vi "Change FPGA Sample Time.vi"(8 "error in":errorcluster, 11 "tCRD in":refnum<class "Aircraft OPCCRD.lvclass">) -> (0 "error out":errorcluster, 3 "tCRD out":refnum<class "Aircraft OPCCRD.lvclass">)   [LabVIEW 2015, in "Aircraft OPCCRD.lvclass"]
uses:
  Aircraft OPCCRD.lvclass
  Reusable/Instrument/Instrument.lvclass/Instrument.ctl
  Aircraft OPCCRD.lvclass/Aircraft OPCCRD.ctl
  Reusable/Instrument/Read Log Session.vi
  Accessors/Read FPGA Ref.vi
  Reusable/Instrument/Write Restart Requested_.vi
  <vilib>/Utility/error.llb/Error Cluster From Error Code.vi
  <vilib>/rvi/errors/niLvFpgaAdjustHostInterfaceError.vi
  <userlib>/_Session Fwk/Session - Root.lvclass
  tFPGA Ref.ctl
  <vilib>/rvi/interface/nirviReadWriteControl/nirviReadWriteControl.xnode
  FPGA Bitfiles/Aircraft OPCRD Server.lvbitx
  Reusable/Instrument/Instrument.lvclass
  Reusable/Session Log/System Log.lvclass
  NiFpgaLv.dll
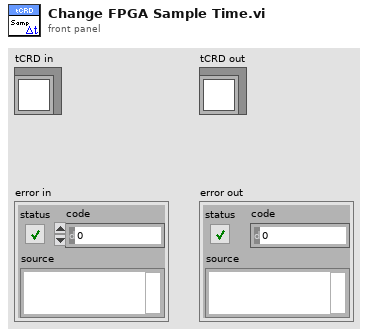
[diagram p1: front panel]
types:
  T1 = typedef "Session - Root.lvclass/Session Handle.ctl" = refnum<data-value>
  T2 = typedef "Aircraft OPCCRD.lvclass/tFPGA Ref.ctl" = refnum<k20>
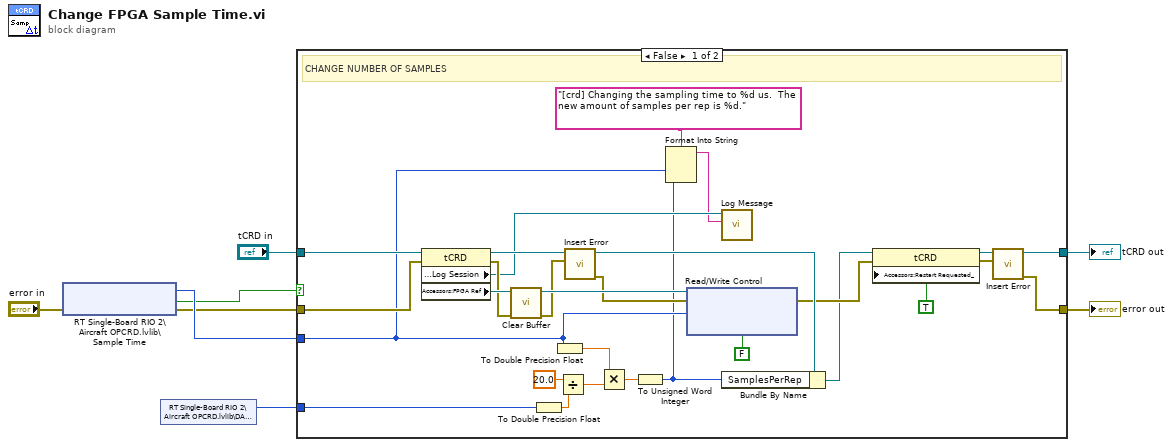
[diagram p0: block diagram]
diagram:
  n1 = shared-variable "RT Single-Board RIO 2\\Aircraft OPCRD.lvlib\\Sample Time"(error in="error in") -> (w8:u16, error out=w5:errorcluster, w2:bool)  [unwired: 1 in]
  n2 = shared-variable "RT Single-Board RIO 2\\Aircraft OPCRD.lvlib\\DAQ Rate"() -> (w1:u8)  [unwired: 1 in, 1 out]
  n3 = case shown="False" w2 {
    tunnel: w5 -> [w15 w38]
    tunnel: "tCRD in" -> [w18 w37]
    tunnel: w8 -> [w12 _]
    tunnel: [w24 w38] -> w6
    tunnel: [w25 w37] -> w3
    tunnel: w1 -> [w33 _]
    frame False {
      # "CHANGE NUMBER OF SAMPLES"
      n4 = property class="tCRD"(reference=w18, error in=w15) -> (reference out=w17:refnum<class "Aircraft OPCCRD.lvclass">, error out=w14:errorcluster, "Accessors:Log Session"=w13:T1, "Accessors:FPGA Ref"=w16:T2)
      n5 = call "Clear Buffer.vi"("error in"=w14, "Refnum in"=w16) -> ("error out"=w28:errorcluster, "FPGA VI Reference Out"=w29:T2)  [unwired: 8 in]
      n6 = To Double Precision Float(number=w33) -> (double precision float=w32:dbl)
      n7 = To Double Precision Float(number=w12) -> (double precision float=w31:dbl)
      n8 = Divide(x=20.0, y=w32) -> (x/y=w35:dbl)
      n9 = call "Insert Error.vi"("err"=w28, "Instrument in"=w17) -> ("error out"=w26:errorcluster, "Instrument out"=w27:refnum<class "Aircraft OPCCRD.lvclass">)  [unwired: 7 in, 1 out]
      n10 = Multiply(x=w31, y=w35) -> (x*y=w36:dbl)
      n11 = To Unsigned Word Integer(number=w36) -> (unsigned 16bit integer=w10:u16)
      n12 = Format Into String(format string="[crd] Changing the sampling time to %d us.  The new amount of samples per rep is %d." ("MSG In"), w12, w10) -> (resulting string=w9:string)  [unwired: 2 in, 1 out]
      n13 = xnode "Read/Write Control"("FPGA VI Reference In"=w29, "error in"=w26, "Sample Time (us)"=w12, "Pause Digitizer"=FALSE) -> ("error out"=w22:errorcluster)  [unwired: 1 out]
      n14 = call "Log Message.vi"("MSG In"=w9, "session in"=w13) -> ()  [unwired: 8 in, 2 out]
      n15 = Bundle By Name(cluster=w27, "SamplesPerRep"=w10) -> (w21:refnum<class "Aircraft OPCCRD.lvclass">)
      n16 = property class="tCRD"(reference=w21, error in=w22, "Accessors:Restart Requested_"=TRUE ("Restart Requested_")) -> (reference out=w20:refnum<class "Aircraft OPCCRD.lvclass">, error out=w19:errorcluster)
      n17 = call "Insert Error.vi"("err"=w19, "Instrument in"=w20) -> ("error out"=w24:errorcluster, "Instrument out"=w25:refnum<class "Aircraft OPCCRD.lvclass">)  [unwired: 7 in, 1 out]
    }
    frame True {
    }
  }
  "error out" <- w6
  "tCRD out" <- w3
